vi "TestMFA.vi"() -> ()   [LabVIEW 2018]
panel:
  out "Homing":bool
  in  "Home":bool
  in  "stop":bool
  out "Camera Position":dbl format="%.2f"
  out "Mirror Position":dbl format="%.2f"
  in  "Axis":u16(ring)=1 items=["Camera"=1, "Mirror"=2]
  out "TimeoutFlag":bool
  in  "Location Setpoint":dbl format="%.2f"
  out "error out":errorcluster
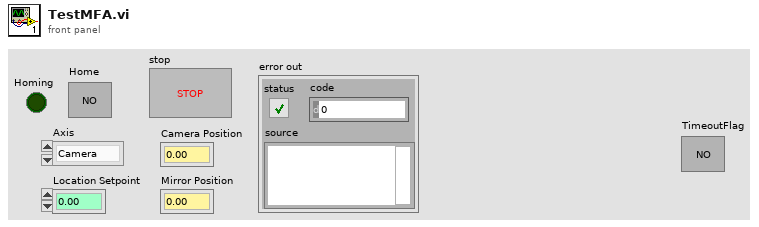
[diagram p1: front panel]
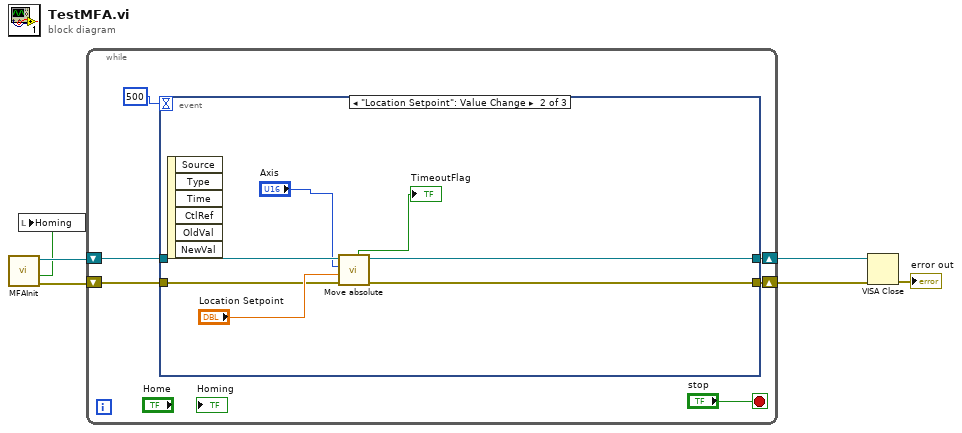
[diagram p0: block diagram]
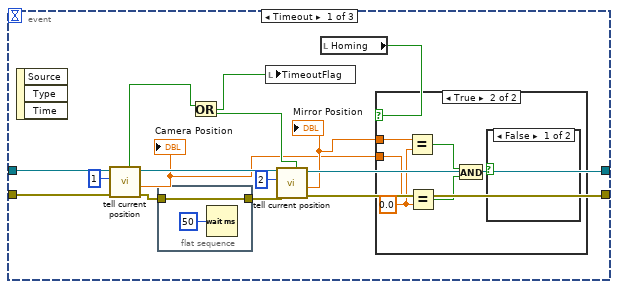
[diagram p2: hidden frame]
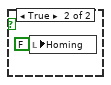
[diagram p4: hidden frame]
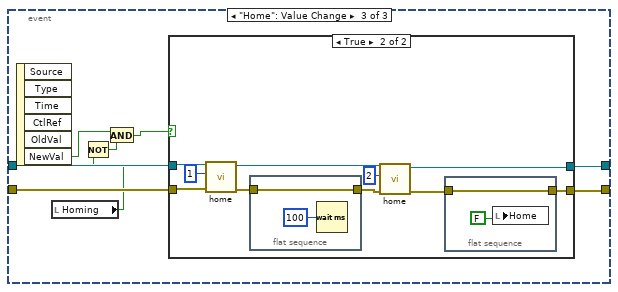
[diagram p5: hidden frame]
diagram:
  n1 = call "MFAInit.vi"() -> ("error out"=w2:errorcluster, "Homing"=w1:bool, "reference out"=w3:refnum<visa-resource-name>)  [unwired: 8 in, 1 out]
  n2 = local write "Homing"(w1) -> ()
  n3 = while {
    shift-right: [w10] -> w4
    shift-left: w2 -> [w9]
    shift-right: [w11] -> w5
    shift-left: w3 -> [w8]
    stop <- "stop" stop-if-true
    n4 = event shown="[1] \"Location Setpoint\": Value Change" {
      selector: _ -> [_ _ _]
      dyn-events: _ -> [_ _ _]
      timeout: 500 -> [_ _ _]
      tunnel: w9 -> [w26 w41 w50]
      tunnel: w8 -> [w27 w42 w51]
      tunnel: [w25 w38 w48] -> w11
      tunnel: [w24 w37 w49] -> w10
      event Timeout {
        n5 = event-data() -> ()  [unwired: 1 in, 3 out]
        n6 = call <instrlib>:"tell current position.vi"("error in"=w26, "Axis in"=1, "VISA Handle in"=w27) -> ("error out"=w17:errorcluster, "Current position (units)"=w13:dbl, "VISA Handle out"=w22:refnum<visa-resource-name>, "TimeoutFlag"=w20:bool)  [unwired: 2 in, 1 out]
        "Camera Position" <- w13
        n7 = flat-sequence {
          tunnel: w17 -> [w36]
          tunnel: [w36] -> w16
          frame #0 {
            n8 = Wait (ms)(milliseconds to wait=u32 50) -> ()  [unwired: 1 out]
          }
        }
        n9 = call <instrlib>:"tell current position.vi"("error in"=w16, "Axis in"=2, "VISA Handle in"=w22) -> ("error out"=w24:errorcluster, "Current position (units)"=w14:dbl, "VISA Handle out"=w25:refnum<visa-resource-name>, "TimeoutFlag"=w19:bool)  [unwired: 2 in, 1 out]
        "Mirror Position" <- w14
        n10 = Or(x=w20, y=w19) -> (x .or. y?=w18:bool)
        n11 = local write "TimeoutFlag"(w18) -> ()
        n12 = local read "Homing"() -> (w15:bool)
        n13 = case shown="True" w15 {
          tunnel: w14 -> [_ w29]
          tunnel: w13 -> [_ w28]
          frame False {
          }
          frame True {
            w30 = 0.0 ("y")
            n14 = Equal?(x=w29, y=w30) -> (x = y?=w33:bool)
            n15 = Equal?(x=w28, y=w30) -> (x = y?=w32:bool)
            n16 = And(x=w33, y=w32) -> (x .and. y?=w31:bool)
            n17 = case shown="False" w31 {
              frame False {
              }
              frame True {
                n18 = local write "Homing"(FALSE ("Homing")) -> ()
              }
            }
          }
        }
      }
      event "Location Setpoint": Value Change {
        n19 = event-data() -> ()  [unwired: 1 in, 6 out]
        n20 = call <instrlib>:"Move absolute.vi"("error in"=w41, "New target position (units)"="Location Setpoint", "Axis in"="Axis", "VISA Handle in"=w42) -> ("error out"=w37:errorcluster, "VISA Handle out"=w38:refnum<visa-resource-name>, "TimeoutFlag"=→"TimeoutFlag":bool)  [unwired: 2 in, 1 out]
      }
      event "Home": Value Change {
        n21 = event-data() -> ("NewVal"=w47:bool)  [unwired: 1 in, 5 out]
        n22 = local read "Homing"() -> (w44:bool)
        n23 = Not(x=w44) -> (.not. x?=w45:bool)
        n24 = And(x=w47, y=w45) -> (x .and. y?=w46:bool)
        n25 = case shown="True" w46 {
          tunnel: w51 -> [w53 w63]
          tunnel: w50 -> [w52 w62]
          tunnel: [w52 w54] -> w49
          tunnel: [w53 w58] -> w48
          frame False {
          }
          frame True {
            n26 = call <instrlib>:"home.vi"("error in"=w62, "Axis in"=1, "VISA Handle in"=w63) -> ("error out"=w61:errorcluster, "VISA Handle out"=w59:refnum<visa-resource-name>)  [unwired: 3 in, 2 out]
            n27 = flat-sequence {
              tunnel: w61 -> [w67]
              tunnel: [w67] -> w57
              frame #0 {
                n28 = Wait (ms)(milliseconds to wait=u32 100) -> ()  [unwired: 1 out]
              }
            }
            n29 = call <instrlib>:"home.vi"("error in"=w57, "Axis in"=2, "VISA Handle in"=w59) -> ("error out"=w55:errorcluster, "VISA Handle out"=w58:refnum<visa-resource-name>)  [unwired: 3 in, 2 out]
            n30 = flat-sequence {
              tunnel: w55 -> [w65]
              tunnel: [w65] -> w54
              frame #0 {
                n31 = local write "Home"(FALSE ("Home")) -> ()
              }
            }
          }
        }
      }
    }
  }
  n32 = VISA Close(VISA resource name=w5, error in (no error)=w4) -> (error out=→"error out":errorcluster)
